vi "Press And Hold Button .vi"(0 "GEA2 Reference In":refnum<k24>, 1 "Delay Time (s)":dbl=3.25 format="%#_13g", 5 "Standalone?":bool, 7 "Button":T2=enum."SW201 - My Cycle", 9 "GEA Inputs":T1 {"Destination" format="%.0x"; "Source" format="%.0x"}, 11 "Error In":errorcluster) -> (4 "GEA2 Reference Out":refnum<k24>, 15 "Error Out":errorcluster)   [LabVIEW 2016, in "TL27.lvlib"]
uses:
  Projects/TL27.lvlib
  type defs/UI Buttons.ctl
  C:/Automation/DLLs/PC Dot Net/GeaCommunication.dll
  Common/LabVIEW GEA2 Toolkit/LabVIEW_GEA2_Toolkit.lvlibp/type defs/Source_Destination.ctl
  Common/LabVIEW GEA2 Toolkit/LabVIEW_GEA2_Toolkit.lvlibp/type defs/ERD Write Data In.ctl
  Common/LabVIEW GEA2 Toolkit/LabVIEW_GEA2_Toolkit.lvlibp/type defs/Data Type.ctl
  Common/LabVIEW GEA2 Toolkit/LabVIEW_GEA2_Toolkit.lvlibp
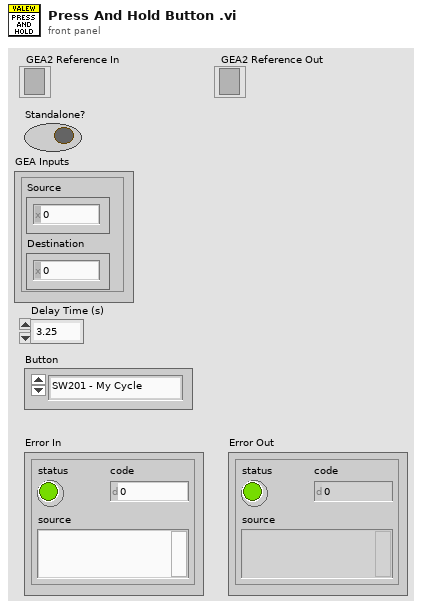
[diagram p1: front panel]
types:
  T1 = typedef "LabVIEW_GEA2_Toolkit.lvlibp/Source_Destination.ctl" = cluster{"Source":u8, "Destination":u8}
  T2 = typedef "TL27.lvlib/UI Buttons.ctl" = enum16{"Switch Off", "SW201 - My Cycle", "SW202 - Delay Wash", "SW203 - Extra Rinse", "SW204 - Signal / Volume", "SW205 - Spin", "SW206 - Deep Rinse / Fab Soft", "SW207 - Soil", "SW208 - Auto Soak", "SW209 - Temp", "SW210 - Warm Rinse", "SW211 - Deep Fill", "SW212 - Stain Remover", "SW213 - Power", "SW222 - Control Lock", "SW214 - Start / Pause", "SW301 - Start/Pause LE", "SW302 - Option Button LE", "SW201/212 - Bulk Flush"}
  T3 = typedef "LabVIEW_GEA2_Toolkit.lvlibp/ERD Write Data In.ctl" = cluster{"ERD Number":u16, "Data Type":T4, "Data":string}
  T4 = typedef "LabVIEW_GEA2_Toolkit.lvlibp/Data Type.ctl" = enum16{"string", "boolean", "uint8_t", "uint16_t", "uint32_t", "uint64_t", "int8_t", "int16_t", "int32_t", "int64_t"}
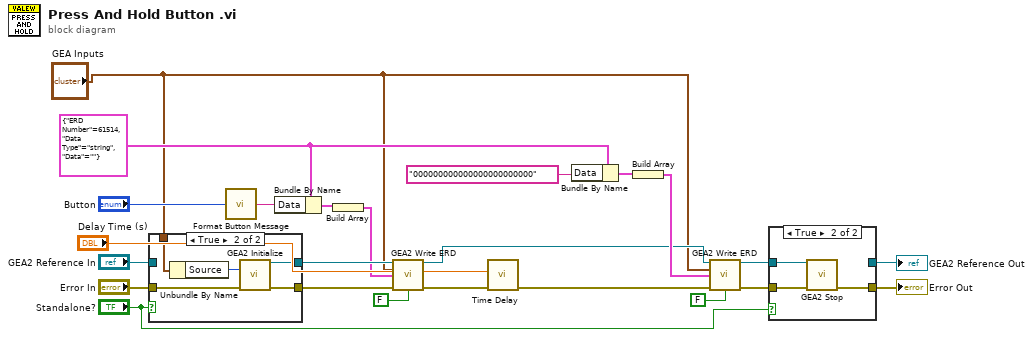
[diagram p0: block diagram]
diagram:
  w4 = T3 {"ERD Number"=61514, "Data Type"=enum."string", "Data"=""} ("ERD Write Data In")
  n1 = case shown="True" "Standalone?" {
    tunnel: "Error In" -> [w25 w31]
    tunnel: [w25 w30] -> w17
    tunnel: "GEA2 Reference In" -> [w26 _]
    tunnel: [w26 w29] -> w15
    tunnel: "GEA Inputs" -> [_ w27]
    frame False {
    }
    frame True {
      n2 = Unbundle By Name(w27) -> ("Source"=w28:u8)
      n3 = call "GEA2 Initialize.vi"("Source Address"=w28, "error in"=w31) -> ("GEA2 Reference Out"=w29:refnum<k24>, "error out"=w30:errorcluster)  [unwired: 11 in, 1 out]
    }
  }
  n4 = call "Format Button Message.vi"("Switch"="Button") -> ("Switch Message"=w14:string)  [unwired: 14 in]
  n5 = Bundle By Name(cluster=w4, "Data"=w14) -> (w13:T3)
  n6 = Build Array(w13) -> (w12:T3[])
  n7 = call "GEA2 Write ERD.vi"("GEA2 Reference In"=w15, "GEA Inputs"="GEA Inputs", "Write ERD List"=w12, "Error In"=w17, "Verify ERD Response?"=FALSE) -> ("GEA2 Reference Out"=w5:refnum<k24>, "Error Out"=w16:errorcluster)  [unwired: 8 in, 1 out]
  n8 = call "Time Delay"("error in (no error)"=w16, "Delay Time (s)"="Delay Time (s)") -> ("error out"=w10:errorcluster)  [unwired: 9 in]
  n9 = Bundle By Name(cluster=w4, "Data"="000000000000000000000000" ("Message")) -> (w7:T3)
  n10 = Build Array(w7) -> (w6:T3[])
  n11 = call "GEA2 Write ERD.vi"("GEA2 Reference In"=w5, "GEA Inputs"="GEA Inputs", "Write ERD List"=w6, "Error In"=w10, "Verify ERD Response?"=FALSE) -> ("GEA2 Reference Out"=w11:refnum<k24>, "Error Out"=w9:errorcluster)  [unwired: 8 in, 1 out]
  n12 = case shown="True" "Standalone?" {
    tunnel: [w32 w36] -> w20
    tunnel: w11 -> [w33 w35]
    tunnel: [w33 _] -> w19
    tunnel: w9 -> [w32 w34]
    frame False {
    }
    frame True {
      n13 = call "GEA2 Stop.vi"("GEA2 Reference In"=w35, "Error In"=w34) -> ("Error Out"=w36:errorcluster)  [unwired: 13 in]
    }
  }
  "Error Out" <- w20
  "GEA2 Reference Out" <- w19
